vi "Get Ingredients.vi"(8 "error in (no error)":errorcluster, 11 "LED Array in":refnum<class "LED Array.lvclass">) -> (0 "error out":errorcluster, 2 "Ingredients":T1[](array[typedef]), 3 "LED Array out":refnum<class "LED Array.lvclass">)   [LabVIEW 2020, in "LED Array.lvclass"]
uses:
  LED Array.lvclass
  Item/Ingredient.ctl
  Item/Item.lvclass
  Electronic Parts/Electronic Parts.lvclass
  C:/dev/IlluminatedG/lv-oopanel-gc-calc/Item/Item.lvclass
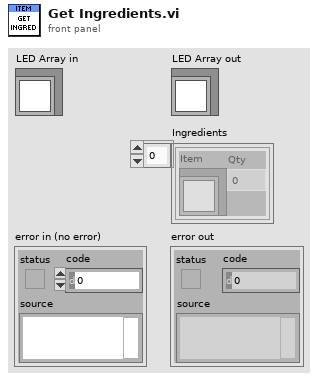
[diagram p1: front panel]
types:
  T1 = typedef "Item.lvclass/Ingredient.ctl" = cluster{"Item":refnum<class "Item.lvclass">, "Qty":dbl}
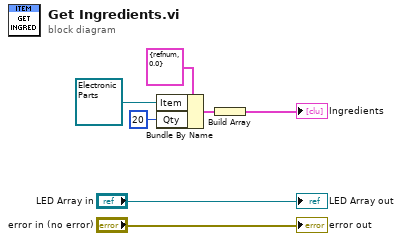
[diagram p0: block diagram]
diagram:
  n1 = Bundle By Name(cluster=T1 {"Item"=refnum, "Qty"=0.0} ("Ingredient"), "Item"=refnum<class "Electronic Parts.lvclass"> refnum ("Electronic Parts.lvclass"), "Qty"=20) -> (w2:T1)
  n2 = Build Array(w2) -> (→"Ingredients":T1[])
  "error out" <- "error in (no error)"
  "LED Array out" <- "LED Array in"
